vi "Teleop Ball V.5.0.vi"   [LabVIEW 2016]
uses:
  <vilib>/Rock Robotics/WPI/Solenoid/WPI_SolenoidValue.ctl
  Robot Global Data V.5.0.vi
  <vilib>/Rock Robotics/WPI/Solenoid/WPI_SolenoidSetEnum.vi
types:
  T1 = typedef "WPI_SolenoidValue.ctl" = enum16{"Off", "On", "Forward", "Reverse"}
  T2 = typedef "WPI_SolenoidDevRef.ctl" = cluster{"DevStatus":errorcluster, "Pneumatics Control Module":u8, "Forward Solenoid Channel":T3, "Reverse Solenoid Channel":T3}
  T3 = typedef "WPI_SolenoidChannel.ctl" = enum8{"Solenoid 0", "Solenoid 1", "Solenoid 2", "Solenoid 3", "Solenoid 4", "Solenoid 5", "Solenoid 6", "Solenoid 7", "Invalid"}
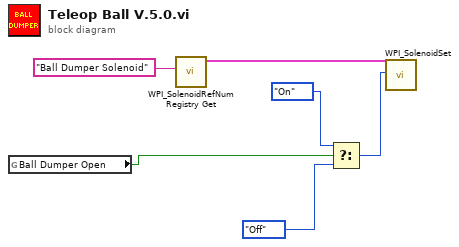
[diagram p0: block diagram]
diagram:
  n1 = global read "Robot Global Data V.5.0.vi" "Ball Dumper Open"() -> (w1:bool)
  n2 = call <vilib>:"WPI_SolenoidRefNum Registry Get.vi"("refnum name"="Ball Dumper Solenoid") -> ("SolenoidDevRef"=w5:T2)  [unwired: 9 in, 1 out]
  n3 = Select(t=WPI_SolenoidValue."On" ("Value"), s=w1, f=WPI_SolenoidValue."Off" ("Value")) -> (s? t:f=w2:T1)
  n4 = call-poly <vilib>:"WPI_SolenoidSet.vi"("Value"=w2, "SolenoidDevRef"=w5) -> ()  [unwired: 8 in, 2 out]
